vi "FEM-03 Test.vi"() -> ()   [LabVIEW 2010, in "FEM-03.lvlib"]
uses:
  FEM-03.lvlib
panel:
  out "GPM":dbl
  in  "stop":bool
  out "error out":errorcluster
  in  "VISA resource name":refnum<visa-resource-name>
  in  "error in":errorcluster
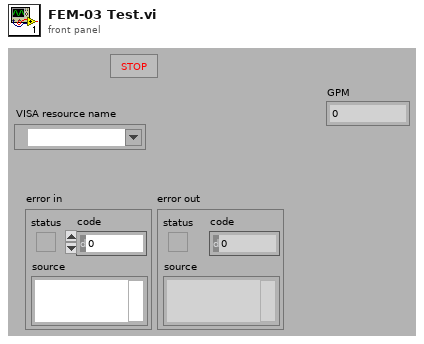
[diagram p1: front panel]
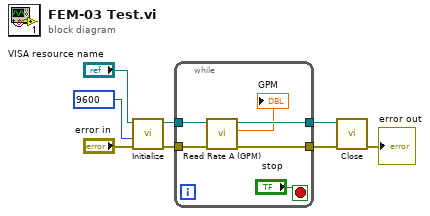
[diagram p0: block diagram]
diagram:
  w2 = u32 9600 items=["9600"=9600, "38400"=38400, "57600"=57600, "19200"=19200] ("Baud Rate")
  n1 = call "Initialize.vi"("error in (no error)"="error in", "Baud Rate"=w2, "VISA resource name"="VISA resource name") -> ("error out"=w5:errorcluster, "VISA resource name out"=w4:refnum<visa-resource-name>)  [unwired: 7 in]
  n2 = while {
    tunnel: w5 -> [w14]
    tunnel: w4 -> [w13]
    tunnel: [w11] -> w3
    tunnel: [w10] -> w1
    stop <- "stop" stop-if-true
    n3 = call "Read Rate A (GPM).vi"("error out"=w14, "VISA resource name out"=w13) -> ("error IO"=w11:errorcluster, "GPM"=→"GPM":dbl, "VISA resource  out"=w10:refnum<visa-resource-name>)  [unwired: 7 in]
  }
  n4 = call "Close.vi"("error in (no error)"=w3, "VISA resource name"=w1) -> ("error out"=→"error out":errorcluster)  [unwired: 9 in]
